vi "Set User Data Folder Internal.vi"(8 "error in (no error)":errorcluster, 10 "User Data":path, 11 "Webview2":refnum<k24>) -> (0 "error out":errorcluster, 3 "Webview2":refnum<k24>)   [LabVIEW 2020, in "WebView2.lvlib" / "WebView2 Control.lvclass"]
uses:
  WebView2 Control.lvclass
  C:/Users/Simon/Documents/GitHub/LV-WebView2/Source/Libs/Microsoft.Web.WebView2.WinForms.dll
  Libs/Microsoft.Web.WebView2.WinForms.dll
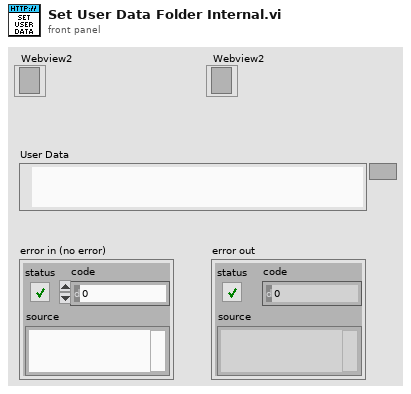
[diagram p1: front panel]
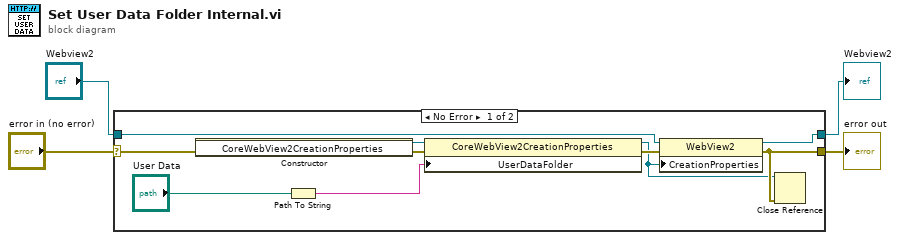
[diagram p0: block diagram]
diagram:
  n1 = case shown="No Error" "error in (no error)" {
    selector: "error in (no error)" -> [w10 w16]
    tunnel: [w14 w15] -> w4
    tunnel: "Webview2" -> [w13 w15]
    tunnel: [w8 w16] -> w1
    frame No Error {
      n2 = constructor class="CoreWebView2CreationProperties"(error in=w10) -> (reference out=w11:refnum<k24>, error out=w9:errorcluster)  [unwired: 2 in, 1 out]
      n3 = Path To String(path="User Data") -> (string=w6:string)
      n4 = property class="CoreWebView2CreationProperties"(reference=w11, error in=w9, "UserDataFolder"=w6) -> (reference out=w7:refnum<k24>, error out=w12:errorcluster)
      n5 = property class="WebView2"(reference=w13, error in=w12, "CreationProperties"=w7) -> (reference out=w14:refnum<k24>, error out=w8:errorcluster)
      n6 = Close Reference(reference=w7, error in (no error)=w8) -> ()  [unwired: 1 out]
    }
    frame Error {
    }
  }
  "error out" <- w1
  "Webview2" <- w4
